vi "MC fill in missing shots in spreadsheet array.vi"(10 "shot #s main":string[](array[string]), 11 "device data in":string[][](array[string])) -> (3 "devive var data out":string[][](array[string]))   [LabVIEW 2020]
panel:
  out "x != y?":bool
  out "size(s)":i32
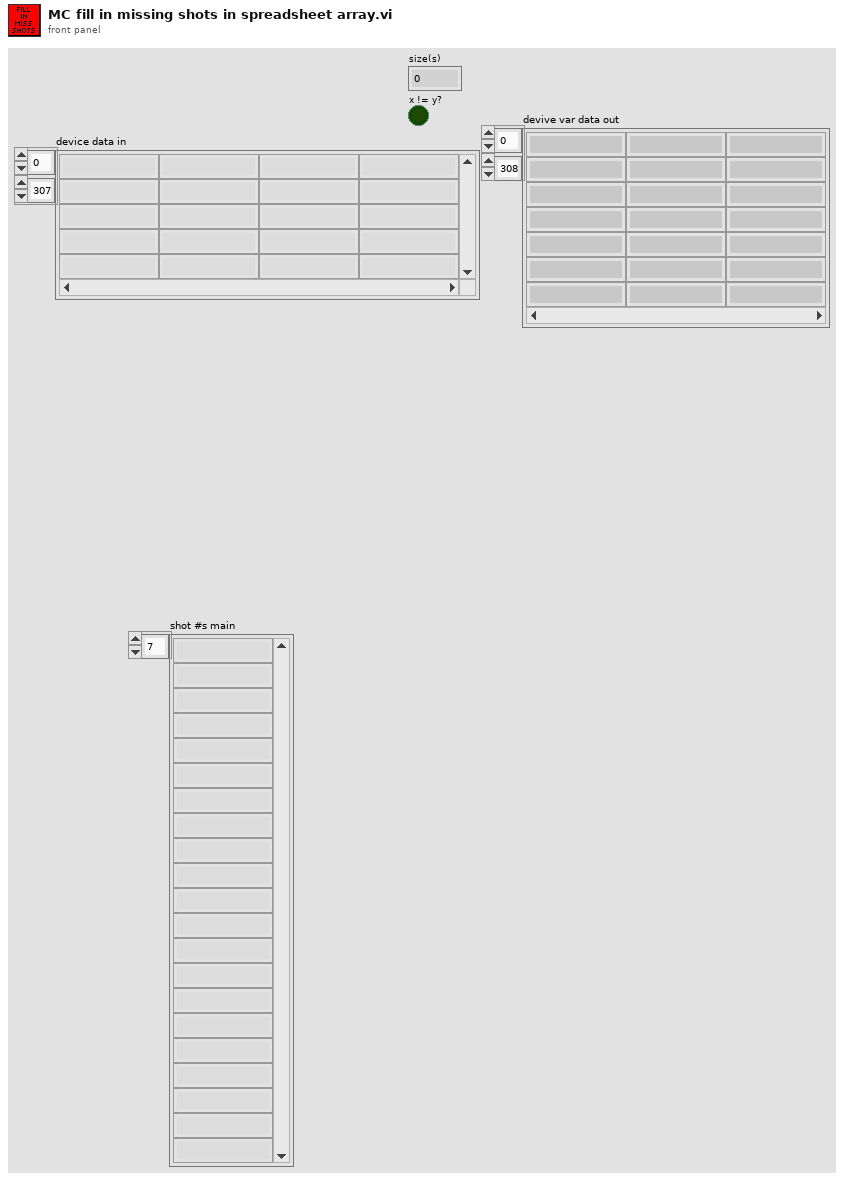
[diagram p1: front panel]
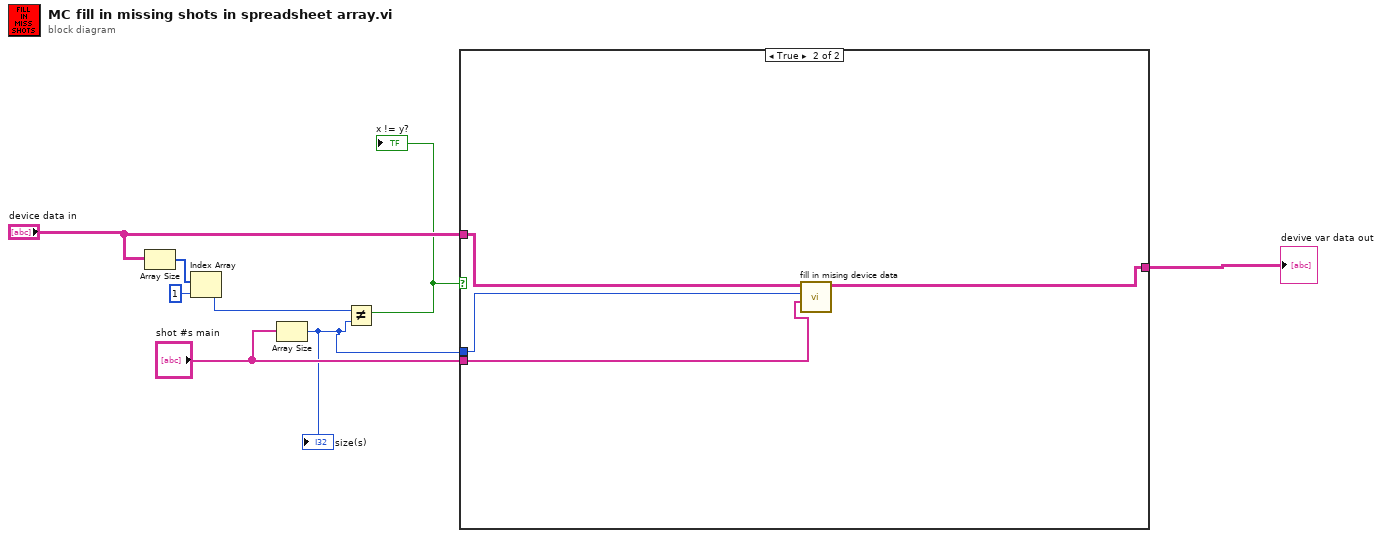
[diagram p0: block diagram]
diagram:
  n1 = Array Size(array="device data in") -> (size(s)=w5:i32[])
  n2 = Index Array(array=w5, index=1) -> (element=w4:i32)
  n3 = Array Size(array="shot #s main") -> (size(s)=w1:i32)
  "size(s)" <- w1
  n4 = Not Equal?(x=w4, y=w1) -> (x != y?=w3:bool)
  "x != y?" <- w3
  n5 = case shown="True" w3 {
    tunnel: "shot #s main" -> [_ w13]
    tunnel: "device data in" -> [w9 w12]
    tunnel: [w9 w11] -> w8
    tunnel: w1 -> [_ w10]
    frame False {
    }
    frame True {
      n6 = call "fill in mising device data.vi"("shot #s main"=w13, "total # shots"=w10, "devive data in"=w12) -> ("Array"=w11:string[][])  [unwired: 8 in]
    }
  }
  "devive var data out" <- w8
